vi "Run_2_of_X_Tests.vi"() -> ()   [LabVIEW 2019]
uses:
  <vilib>/Rock Robotics/WPI/ThirdParty/JAS_Junk/TrajLib/Trajectory_Library.lvlib
panel:
  out "Meca Drive \nPose Est 2":bool
  out "Meca Drive \nPose Est":bool
  out "Meca Drive \nOdometry":bool
  out "Meca Drive \nKinematics":bool
  out "String":string
  out "Flywheel Simulation":bool
  out "Matrix":bool
  out "PID":bool
  out "Math Utils":bool
  out "Linear Filter":bool
  out "Linear System Loop":bool
  out "All Tests Finished":bool
  out "Holonomic Drive Ctrl":bool
  out "Linear Plant Inv FF":bool
  out "Numerical Jacobian":bool
  out "Merwe Scaled Sigma Pts":bool
  out "Numerical Integration":bool
  out "Median Filter":bool
  out "Linear System ID":bool
  out "Kalman filter":bool
  out "PID Input / Output":bool
  out "Linear Quadradtic Regulator":bool
  # "FORMAL TRAJECTORY / CONTROL LIBRARY TEST PROCEDURE"
  # "FUNCTION NOT\nIMPLEMENTED"
  # "Extended Kalman Filter"
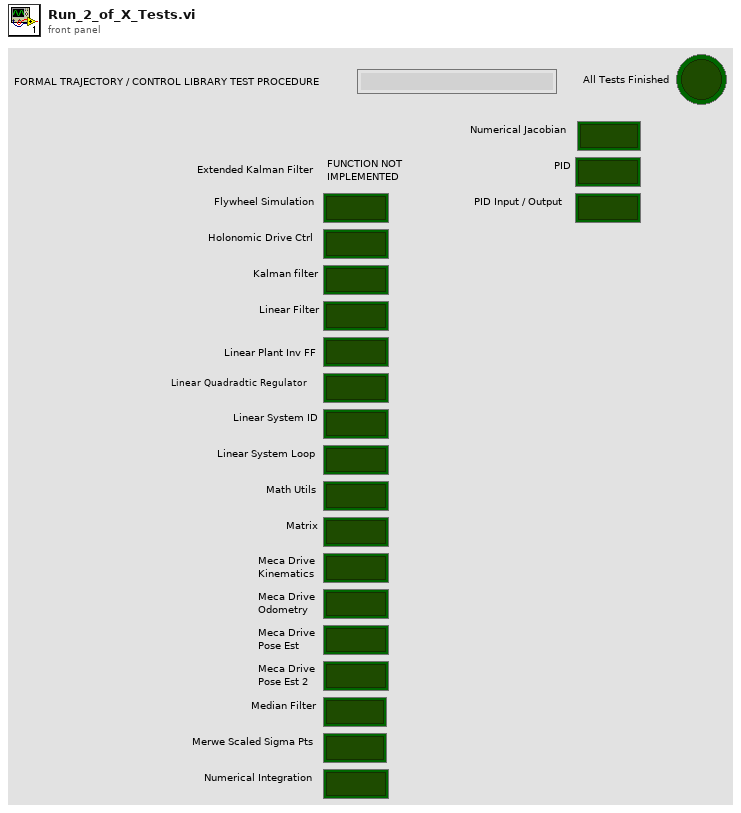
[diagram p1: front panel]
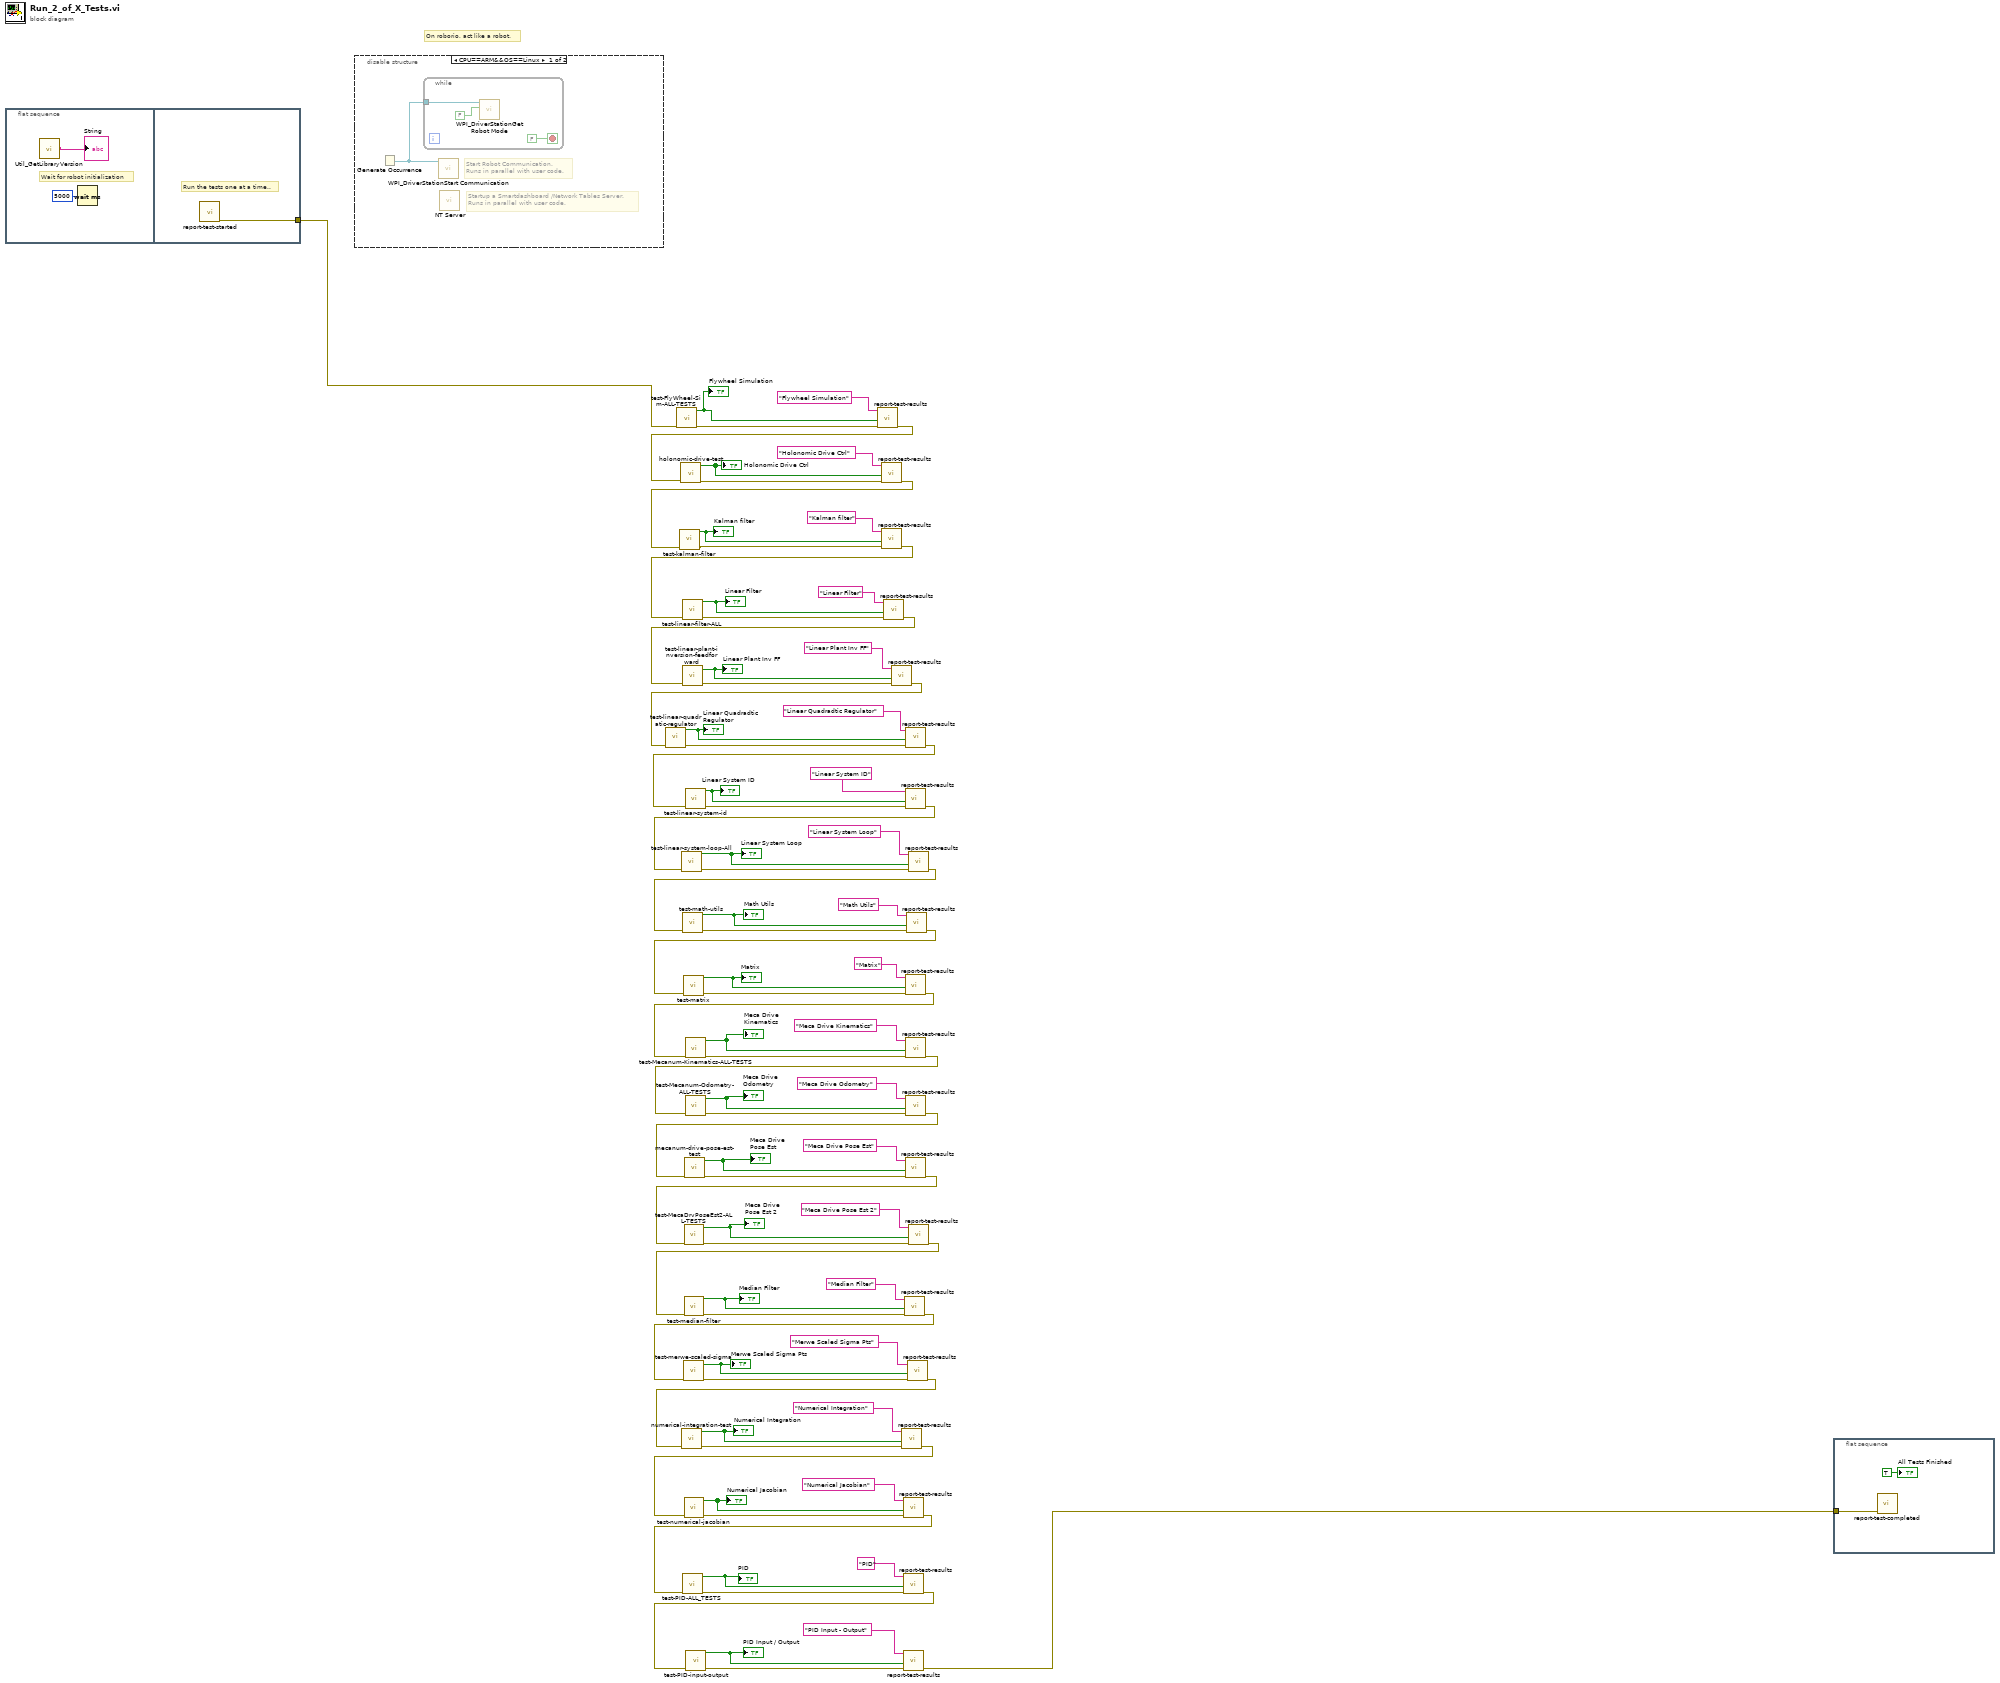
[diagram p0: block diagram]
diagram:
  # "On roborio, act like a robot."
  n1 = flat-sequence {
    tunnel: [w84] -> w6
    frame #0 {
      # "Wait for robot initialization"
      n2 = call <vilib>:"Util_GetLibraryVersion.vi"() -> ("TrajLibVersion"=→"String":string)  [unwired: 11 in]
      n3 = Wait (ms)(milliseconds to wait=u32 5000) -> ()  [unwired: 1 out]
    }
    frame #1 {
      # "Run the tests one at a time.."
      n4 = call "report-test-started.vi"() -> ("error out"=w84:errorcluster)  [unwired: 11 in]
    }
  }
  n5 = disable-structure shown="CPU==ARM&&OS==Linux" {
    frame condition #0 {
      # "Startup a Smartdashboard /Network Tables Server.\nRuns in parallel with user code."
      # "Start Robot Communication.\nRuns in parallel with user code."
      n6 = Generate Occurrence() -> (w85:refnum<k4>)
      n7 = while {
        tunnel: w85 -> [w88]
        stop <- FALSE stop-if-true
        n8 = call <vilib>:"WPI_DriverStationGet Robot Mode.vi"("Finish"=FALSE, "DS Occurrence"=w88) -> ()  [unwired: 10 out]
      }
      n9 = call <vilib>:"WPI_DriverStationStart Communication.vi"("occurrence"=w85) -> ()  [unwired: 2 in, 9 out]
      n10 = call <vilib>:"NT Server.vi"() -> ()  [unwired: 11 in, 1 out]
    }
    frame condition #1 (active) {
    }
  }
  n11 = call "test-FlyWheel-Sim-ALL-TESTS.vi"("error in (no error)"=w6) -> ("error out"=w21:errorcluster, "All Passed"=w19:bool)  [unwired: 9 in]
  "Flywheel Simulation" <- w19
  n12 = call "report-test-results.vi"("error in (no error)"=w21, "TestPassed"=w19, "Test Name"="Flywheel Simulation") -> ("error out"=w20:errorcluster)  [unwired: 8 in]
  n13 = call "holonomic-drive-test.vi"("error in (no error)"=w20) -> ("error out"=w51:errorcluster, "ALL TESTS PASSED"=w79:bool)  [unwired: 9 in]
  "Holonomic Drive Ctrl" <- w79
  n14 = call "report-test-results.vi"("error in (no error)"=w51, "TestPassed"=w79, "Test Name"="Holonomic Drive Ctrl") -> ("error out"=w50:errorcluster)  [unwired: 8 in]
  n15 = call "test-kalman-filter.vi"("error in (no error)"=w50) -> ("error out"=w49:errorcluster, "ALL TESTS PASSED"=w78:bool)  [unwired: 9 in]
  "Kalman filter" <- w78
  n16 = call "report-test-results.vi"("error in (no error)"=w49, "TestPassed"=w78, "Test Name"="Kalman filter") -> ("error out"=w48:errorcluster)  [unwired: 8 in]
  n17 = call "test-linear-filter-ALL.vi"("error in (no error)"=w48) -> ("error out"=w46:errorcluster, "ALL TESTS GOOD"=w69:bool)  [unwired: 9 in]
  "Linear Filter" <- w69
  n18 = call "report-test-results.vi"("error in (no error)"=w46, "TestPassed"=w69, "Test Name"="Linear Filter") -> ("error out"=w45:errorcluster)  [unwired: 8 in]
  n19 = call "test-linear-plant-inversion-feedforward.vi"("error in (no error)"=w45) -> ("error out"=w44:errorcluster, "All Tests Passed"=w68:bool)  [unwired: 9 in]
  "Linear Plant Inv FF" <- w68
  n20 = call "report-test-results.vi"("error in (no error)"=w44, "TestPassed"=w68, "Test Name"="Linear Plant Inv FF") -> ("error out"=w43:errorcluster)  [unwired: 8 in]
  n21 = call "test-linear-quadratic-regulator.vi"("error in (no error)"=w43) -> ("error out"=w42:errorcluster, "ALL TESTS GOOD"=w67:bool)  [unwired: 9 in]
  "Linear Quadradtic Regulator" <- w67
  n22 = call "report-test-results.vi"("error in (no error)"=w42, "TestPassed"=w67, "Test Name"="Linear Quadradtic Regulator") -> ("error out"=w41:errorcluster)  [unwired: 8 in]
  n23 = call "test-linear-system-id.vi"("error in (no error)"=w41) -> ("error out"=w40:errorcluster, "All tests passed"=w66:bool)  [unwired: 9 in]
  "Linear System ID" <- w66
  n24 = call "report-test-results.vi"("error in (no error)"=w40, "TestPassed"=w66, "Test Name"="Linear System ID") -> ("error out"=w32:errorcluster)  [unwired: 8 in]
  n25 = call "test-linear-system-loop-All.vi"("error in (no error)"=w32) -> ("error out"=w33:errorcluster, "ALL TEsts Passed"=w65:bool)  [unwired: 9 in]
  "Linear System Loop" <- w65
  n26 = call "report-test-results.vi"("error in (no error)"=w33, "TestPassed"=w65, "Test Name"="Linear System Loop") -> ("error out"=w31:errorcluster)  [unwired: 8 in]
  n27 = call "test-math-utils.vi"("error in (no error)"=w31) -> ("error out"=w30:errorcluster, "ALL TESTS PASSED"=w64:bool)  [unwired: 9 in]
  "Math Utils" <- w64
  n28 = call "report-test-results.vi"("error in (no error)"=w30, "TestPassed"=w64, "Test Name"="Math Utils") -> ("error out"=w29:errorcluster)  [unwired: 8 in]
  n29 = call "test-matrix.vi"("error in (no error)"=w29) -> ("error out"=w34:errorcluster, "All Tests\nPassed"=w63:bool)  [unwired: 9 in]
  "Matrix" <- w63
  n30 = call "report-test-results.vi"("error in (no error)"=w34, "TestPassed"=w63, "Test Name"="Matrix") -> ("error out"=w15:errorcluster)  [unwired: 8 in]
  n31 = call "test-Mecanum-Kinematics-ALL-TESTS.vi"("error in (no error)"=w15) -> ("error out"=w17:errorcluster, "All Passed"=w16:bool)  [unwired: 9 in]
  "Meca Drive \nKinematics" <- w16
  n32 = call "report-test-results.vi"("error in (no error)"=w17, "TestPassed"=w16, "Test Name"="Meca Drive Kinematics") -> ("error out"=w11:errorcluster)  [unwired: 8 in]
  n33 = call "test-Mecanum-Odometry-ALL-TESTS.vi"("error in (no error)"=w11) -> ("error out"=w13:errorcluster, "All Passed"=w12:bool)  [unwired: 9 in]
  "Meca Drive \nOdometry" <- w12
  n34 = call "report-test-results.vi"("error in (no error)"=w13, "TestPassed"=w12, "Test Name"="Meca Drive Odometry") -> ("error out"=w7:errorcluster)  [unwired: 8 in]
  n35 = call "mecanum-drive-pose-est-test.vi"("error in (no error)"=w7) -> ("error out"=w9:errorcluster, "Test Passed"=w8:bool)  [unwired: 9 in]
  "Meca Drive \nPose Est" <- w8
  n36 = call "report-test-results.vi"("error in (no error)"=w9, "TestPassed"=w8, "Test Name"="Meca Drive Pose Est") -> ("error out"=w2:errorcluster)  [unwired: 8 in]
  n37 = call "test-MecaDrvPoseEst2-ALL-TESTS.vi"("error in (no error)"=w2) -> ("error out"=w4:errorcluster, "All Passed"=w3:bool)  [unwired: 9 in]
  "Meca Drive \nPose Est 2" <- w3
  n38 = call "report-test-results.vi"("error in (no error)"=w4, "TestPassed"=w3, "Test Name"="Meca Drive Pose Est 2") -> ("error out"=w1:errorcluster)  [unwired: 8 in]
  n39 = call "test-median-filter.vi"("error in (no error)"=w1) -> ("error out"=w35:errorcluster, "ALL TESTS PASSED"=w62:bool)  [unwired: 9 in]
  "Median Filter" <- w62
  n40 = call "report-test-results.vi"("error in (no error)"=w35, "TestPassed"=w62, "Test Name"="Median Filter") -> ("error out"=w28:errorcluster)  [unwired: 8 in]
  n41 = call "test-merwe-scaled-sigma.vi"("error in (no error)"=w28) -> ("error out"=w36:errorcluster, "All Tests Passed"=w52:bool)  [unwired: 9 in]
  "Merwe Scaled Sigma Pts" <- w52
  n42 = call "report-test-results.vi"("error in (no error)"=w36, "TestPassed"=w52, "Test Name"="Merwe Scaled Sigma Pts") -> ("error out"=w27:errorcluster)  [unwired: 8 in]
  n43 = call "numerical-integration-test.vi"("error in (no error)"=w27) -> ("error out"=w37:errorcluster, "All passed"=w53:bool)  [unwired: 9 in]
  "Numerical Integration" <- w53
  n44 = call "report-test-results.vi"("error in (no error)"=w37, "TestPassed"=w53, "Test Name"="Numerical Integration") -> ("error out"=w26:errorcluster)  [unwired: 8 in]
  n45 = call "test-numerical-jacobian.vi"("error in (no error)"=w26) -> ("error out"=w38:errorcluster, "ALL Tests Passed"=w54:bool)  [unwired: 9 in]
  "Numerical Jacobian" <- w54
  n46 = call "report-test-results.vi"("error in (no error)"=w38, "TestPassed"=w54, "Test Name"="Numerical Jacobian") -> ("error out"=w25:errorcluster)  [unwired: 8 in]
  n47 = call "test-PID-ALL_TESTS.vi"("error in (no error)"=w25) -> ("error out"=w39:errorcluster, "All Passed"=w55:bool)  [unwired: 9 in]
  "PID" <- w55
  n48 = call "report-test-results.vi"("error in (no error)"=w39, "TestPassed"=w55, "Test Name"="PID") -> ("error out"=w24:errorcluster)  [unwired: 8 in]
  n49 = call "test-PID-input-output.vi"("error in (no error)"=w24) -> ("error out"=w47:errorcluster, "All Passed"=w56:bool)  [unwired: 9 in]
  "PID Input / Output" <- w56
  n50 = call "report-test-results.vi"("error in (no error)"=w47, "TestPassed"=w56, "Test Name"="PID Input - Output") -> ("error out"=w23:errorcluster)  [unwired: 8 in]
  n51 = flat-sequence {
    tunnel: w23 -> [w89]
    frame #0 {
      n52 = call "report-test-completed.vi"("error in (no error)"=w89) -> ()  [unwired: 10 in, 1 out]
      "All Tests Finished" <- TRUE ("All Tests Finished")
    }
  }
